vi "Find FIFO Indexes.vi"(8 "error in":errorcluster, 10 "Item Name":string, 11 "Custom Device Ref in":T1 format="%.0x") -> (0 "error out":errorcluster, 3 "Index":i32)   [LabVIEW 2020, in "Regatron G5 Custom Device Engine.lvlib"]
uses:
  <vilib>/NI VeriStand/Custom Device API/Custom Device Item Ref.ctl
  Regatron G5 Custom Device Engine.lvlib
  <vilib>/NI VeriStand/Custom Device API/Custom Device API.lvlib
  <vilib>/NI VeriStand/Custom Device Tools/Custom Device Utility Library/Custom Device Utility Library.lvlib
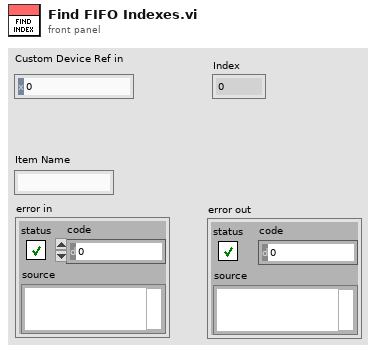
[diagram p1: front panel]
types:
  T1 = typedef "Custom Device API.lvlib/Custom Device Item Ref.ctl" = u64
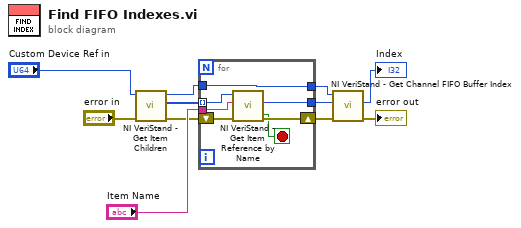
[diagram p0: block diagram]
diagram:
  n1 = call <vilib>:"NI VeriStand - Get Item Children.vi"("error in (no error)"="error in", "Item Ref in"="Custom Device Ref in") -> ("error out"=w4:errorcluster, "Child Refs"=w5:T1[], "Item Ref out"=w2:T1)  [unwired: 6 in, 1 out]
  n2 = for {
    tunnel: [w18] -> w11
    tunnel: "Item Name" -> [w16]
    shift-right: [w17] -> w9
    shift-left: w4 -> [w15]
    tunnel: w5 -> [w14] mode=indexing
    tunnel: w2 -> [w12]
    tunnel: [w12] -> w1
    stop <- w13 stop-if-true
    n3 = call <vilib>:"NI VeriStand - Get Item Reference by Name.vi"("error in (no error)"=w15, "Item Name"=w16, "Parent Ref in"=w14) -> ("error out"=w17:errorcluster, "Item Ref"=w18:T1, "Found"=w13:bool)  [unwired: 5 in, 1 out]
  }
  n4 = call <vilib>:"NI VeriStand - Get Channel FIFO Buffer Index.vi"("error in"=w9, "Channel Ref"=w11, "Device Ref in"=w1) -> ("error out"=→"error out":errorcluster, "Channel FIFO Buffer Index"=→"Index":i32)  [unwired: 4 in, 3 out]
